vi "BS find the buoys.vi"(0 "Image Path":T1, 2 "templete path":string="buoy templete.png", 3 "error in":errorcluster) -> (5 "Matches":T2(array[cluster]) {"Bounding Box"."y" format="%.2f"; "Bounding Box"."x" format="%.2f"; "Position"."y" format="%.2f"; "Position"."x" format="%.2f"; "Score" format="%.2f"; "Scale" format="%.2f"; "Angle" format="%.2f"}, 6 "Valid?":bool, 7 "error out":errorcluster)   [LabVIEW 2012]
doc: "This VI will find up to (4) buoys. It accepts the pool image and the templete image for the buoy. The output is an array of buoy positions in X and Y. The valid? line indicates the tug was found."
uses:
  <vilib>/vision/Image Controls.llb/IMAQ Image.ctl
panel:
  out "Templete Image":T1(plugin-control)
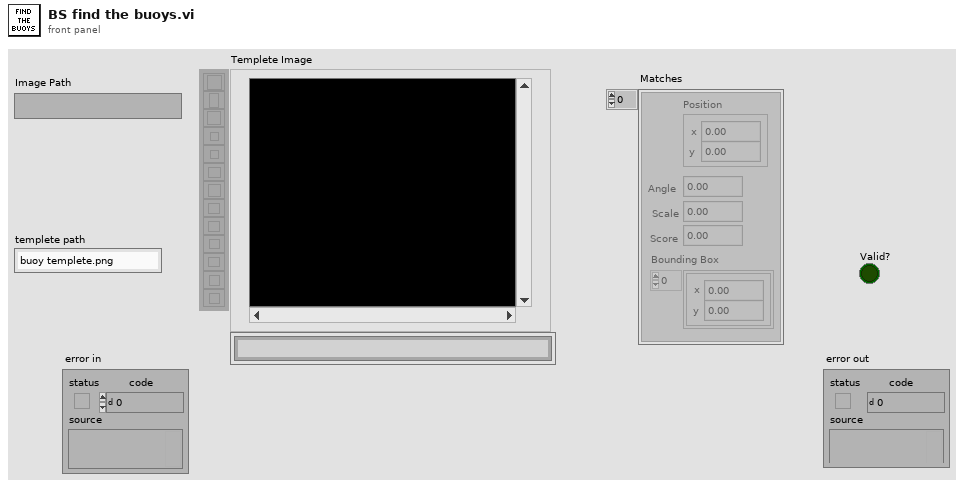
[diagram p1: front panel]
types:
  T1 = typedef "IMAQ Image.ctl" = refnum<image>
  T2 = cluster{"Position":cluster{"x":sgl, "y":sgl}, "Angle":sgl, "Scale":sgl, "Score":sgl, "Bounding Box":cluster{"x":sgl, "y":sgl}[]}[]
  T3 = cluster{"Global Rectangle":i32[], "Contours":cluster{"ID":enum32{"External", "Internal"}, "Type":u32, "Coordinates":i32[]}[]}
  T4 = typedef "Image Type" = u32
  T5 = cluster{"Match Mode (Pattern Matching 1)":u16, "Subpixel Accuracy (Pattern Matching 1)":bool, "Rotation Angle Ranges (degrees) (Pattern Matching 1)":cluster{sgl, sgl}[]}
  T6 = cluster{"ROI Descriptor (Pattern Matching 1)":cluster{"Global Rectangle":i32[], "Contours":cluster{"ID":enum32{"External", "Internal"}, "Type":u32, "Coordinates":i32[]}[]}, "Number of Matches Requested (Pattern Matching 1)":i32, "Minimum Match Score (Pattern Matching 1)":sgl}
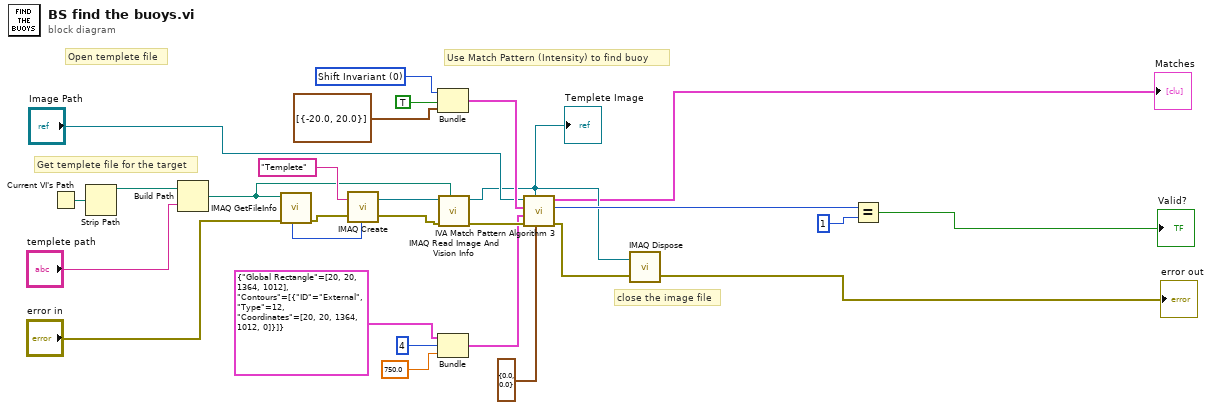
[diagram p0: block diagram]
diagram:
  w28 = u16 0 items=["Shift Invariant", "Rotation Invariant"] ("Match Mode (Pattern Matching 1)")
  # "close the image file"
  # "Use Match Pattern (Intensity) to find buoy"
  # "Open templete file"
  # "Get templete file for the target"
  n1 = Current VI's Path() -> (path=w21:path)
  n2 = Strip Path(path=w21) -> (stripped path=w20:path)  [unwired: 1 out]
  n3 = Build Path(base path=w20, name or relative path="templete path") -> (appended path=w16:path)
  n4 = call "IMAQ GetFileInfo"("error in (no error)"="error in", "File Path"=w16) -> ("error out"=w19:errorcluster, "Image Type"=w18:T4)  [unwired: 3 in, 5 out]
  n5 = call "IMAQ Create"("Image Name"="Templete", "Image Type"=w18, "error in (no error)"=w19) -> ("New Image"=w14:T1, "error out"=w15:errorcluster)  [unwired: 1 in, 1 out]
  n6 = Bundle("Match Mode (Pattern Matching 1)"=w28, "Subpixel Accuracy (Pattern Matching 1)"=TRUE, "Rotation Angle Ranges (degrees) (Pattern Matching 1)"=cluster{sgl, sgl}[] [{-20.0, 20.0}]) -> (w11:T5)  [unwired: 1 out]
  n7 = Bundle("ROI Descriptor (Pattern Matching 1)"=T3 {"Global Rectangle"=[20, 20, 1364, 1012], "Contours"=[{"ID"=enum."External", "Type"=12, "Coordinates"=[20, 20, 1364, 1012, 0]}]}, "Number of Matches Requested (Pattern Matching 1)"=4, "Minimum Match Score (Pattern Matching 1)"=sgl 750.0) -> (w12:T6)  [unwired: 1 out]
  n8 = call "IMAQ Read Image And Vision Info"("File Path"=w16, "error in (no error)"=w15, "Image"=w14) -> ("error out"=w13:errorcluster, "Image Out"=w2:T1)  [unwired: 1 in, 6 out]
  "Templete Image" <- w2
  n9 = call <vilib>:"IVA Match Pattern Algorithm 3.vi"("Match Offset"=cluster{"X":sgl, "Y":sgl} {"X"=0.0, "Y"=0.0} ("Match Offset (Pattern Matching 1)"), "Image Template"=w2, "error in (no error)"=w13, "Match Parameters"=w12, "Setup Match Parameters"=w11, "Image"="Image Path") -> ("error out"=w6:errorcluster, "Number of Matches"=w10:i32, "Matches"=→"Matches":T2)  [unwired: 3 out]
  n10 = call "IMAQ Dispose"("Image"=w2, "error in (no error)"=w6) -> ("error out"=→"error out":errorcluster)  [unwired: 4 in]
  n11 = Equal?(x=w10, y=1) -> (x = y?=→"Valid?":bool)
